vi "CH_LM Config Display.vi"(0 "Meter Index":i32, 1 "Contrast (0.5)":dbl=0.5, 3 "Text (empty)":string, 4 "Clear (false)":bool, 5 "error in (no error)":errorcluster, 7 "Timeout / ms (3000)":i32=3000, 8 "Action (query)":bool, 9 "Lock Timeout / ms (1000)":i32=1000) -> (11 "Lock timed out":bool, 14 "Meter Index":i32, 15 "Contrast":dbl, 19 "error out":errorcluster)   [LabVIEW 2012, in "CH_LM.lvlib"]
doc: "This command will set the display contrast and text in the measurement display area. This command should also be used to clear dismissible error displays on the LCD.\n\nWhen text is displayed through the host interface, it will remain until it is cleared from the front panel, changed again from the host interface, or until a display clear is sent. \n\nThe amount of text that can be displayed will be limited to TBD. \n\n<B>Hint:</B> The string will be displayed centered. Oversized strings are left and right truncated. All text within the quoted string will be displayed."
uses:
  CH_LM.lvlib
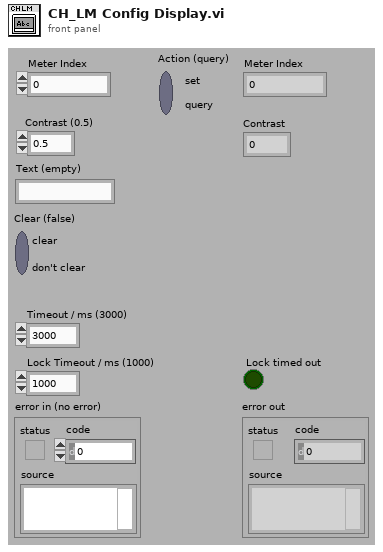
[diagram p1: front panel]
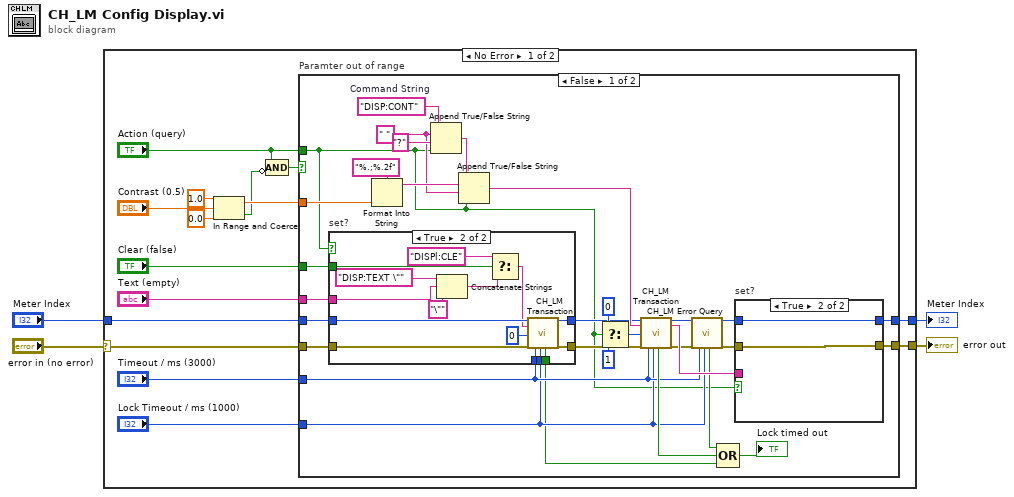
[diagram p0: block diagram]
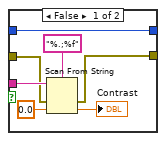
[diagram p3: hidden frame]
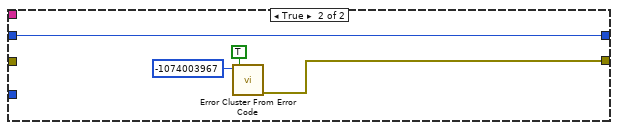
[diagram p4: hidden frame]
diagram:
  n1 = case shown="No Error" "error in (no error)" {
    selector: "error in (no error)" -> [w19 w82]
    tunnel: [w17 w82] -> w4
    tunnel: "Meter Index" -> [w18 w81]
    tunnel: [w16 w81] -> w1
    frame No Error {
      n2 = In Range and Coerce(upper limit=1.0, x="Contrast (0.5)", lower limit=0.0) -> (coerced(x)=w13:dbl, In Range?=w10:bool)
      n3 = Compound Arithmetic op=AND("Action (query)", invert w10) -> (w8:bool)
      n4 = case "Paramter out of range" shown="False" w8 {
        tunnel: w19 -> [w27 _]
        tunnel: w18 -> [w28 w80]
        tunnel: [w48 w78] -> w17
        tunnel: [w42 w80] -> w16
        tunnel: "Timeout / ms (3000)" -> [w23 _]
        tunnel: "Lock Timeout / ms (1000)" -> [w22 _]
        tunnel: w13 -> [w34 _]
        tunnel: "Action (query)" -> [w20 _]
        tunnel: "Clear (false)" -> [w29 _]
        tunnel: "Text (empty)" -> [w24 _]
        frame False {
          w32 = " "
          w50 = "DISP:CONT"  # Command String
          n5 = case "set?" shown="True" w20 {
            tunnel: w29 -> [_ w67]
            tunnel: w28 -> [w52 w66]
            tunnel: w27 -> [w51 w65]
            tunnel: [w52 w64] -> w26
            tunnel: [w51 w63] -> w25
            tunnel: w24 -> [_ w58]
            tunnel: w23 -> [_ w55]
            tunnel: w22 -> [_ w54]
            tunnel: [_ w53] -> w21
            frame False {
            }
            frame True {
              n6 = Concatenate Strings("DISP:TEXT \"" ("Command String"), w58, "\"" ("string")) -> (w56:string)
              n7 = Select(t="DISPl:CLE" ("Command String"), s=w67, f=w56) -> (s? t:f=w61:string)
              n8 = call "CH_LM Transaction.vi"("Meter Index"=w66, "Command String"=w61, "NofStrings (-1:all)"=0, "error in (no error)"=w65, "Timeout / ms (3000)"=w55, "Lock Timeout / ms (1000)"=w54) -> ("Lock timed out"=w53:bool, "Meter Index"=w64:i32, "error out"=w63:errorcluster)  [unwired: 11 out]
            }
          }
          n9 = Format Into String(format string="%.;%.2f", w34) -> (resulting string=w33:string)  [unwired: 2 in, 1 out]
          n10 = Append True/False String(1:w20, 2:"?" ("true string"), 3:w32, 4:w50) -> (0:w31:string)
          n11 = Append True/False String(1:w20, 2:w32, 3:w33, 4:w31) -> (0:w30:string)
          n12 = Select(t=0, s=w20, f=1 ("NofStrings (-1:all)")) -> (s? t:f=w44:i32)
          n13 = call "CH_LM Transaction.vi"("Meter Index"=w26, "Command String"=w30, "NofStrings (-1:all)"=w44, "error in (no error)"=w25, "Timeout / ms (3000)"=w23, "Lock Timeout / ms (1000)"=w22) -> ("Lock timed out"=w36:bool, "Meter Index"=w41:i32, "Response"=w49:string, "error out"=w39:errorcluster)  [unwired: 10 out]
          n14 = call "CH_LM Error Query.vi"("Meter Index"=w41, "error in (no error)"=w39, "Timeout / ms (3000)"=w23, "Lock Timeout / ms (1000)"=w22) -> ("Lock timed out"=w37:bool, "Meter Index"=w40:i32, "error out"=w38:errorcluster)  [unwired: 13 out]
          n15 = Compound Arithmetic op=OR(w37, w36, w21) -> (→"Lock timed out":bool)
          n16 = case "set?" shown="True" w20 {
            tunnel: w49 -> [w74 _]
            tunnel: w38 -> [w73 w76]
            tunnel: [w72 w76] -> w48
            tunnel: w40 -> [w69 w75]
            tunnel: [w69 w75] -> w42
            frame False {
              n17 = Scan From String(format string="%.;%f", input string=w74, error in=w73, default 1=0.0 ("default value 1")) -> (error out=w72:errorcluster, output 1=→"Contrast":dbl)  [unwired: 1 in, 2 out]
            }
            frame True {
            }
          }
        }
        frame True {
          n18 = call <vilib>:"Error Cluster From Error Code.vi"("show call chain? (False)"=TRUE, "error code (0)"=-1074003967) -> ("error out"=w78:errorcluster)  [unwired: 1 in, 6 out]
        }
      }
    }
    frame Error {
    }
  }
  "error out" <- w4
  "Meter Index" <- w1
